vi "USG_Query HW.vi"(0 "System no.":i32=1 min=1 max=4 step=1, 5 "error in":errorcluster) -> (14 "List of Hardware Overview":string, 19 "error out":errorcluster)   [LabVIEW 2020]
doc: "USG? HW (Hardware Overview)\n\nDescription\nOutputs the \"HW\" section of the user guide. The \"HW\" section contains information on the \ncurrent hardware configuration and the associated firmware.\n\nFormat\nUSG? HW\n\nArguments\nnone\n\nResponse\nUSG? HW outputs a list of information on the hardware and firmware of the controller. The \nresponse consists of a block:\nThe HW block consists of at least the following fields:\n- Matchcode Match code of the hardware\n- Version Version of the hardware\n- Serial Number Serial number of the hardware\n- Date Production date of the hardware\nIn addition, the HW block contains at least the subblocks Dynamic HW and FW: \nThe Dynamic HW block consists of at least the following fields:\n- Property A property of the hardware, e.g. MAC address or vendor ID \n- Type Data type of the property value\n- Value Property value\nThe FW block consists of at least the following fields:\n- Container Unit Alias for the container unit to which the firmware belongs\n- Function Unit Alias for the function unit to which the firmware belongs\n- ID Index of the firmware in the controller\n- Matchcode Match code of the firmware\n- Version Version of the firmware\n- Date Date of the firmware\n- Compatibility Compatibility index\n- Description Short description of the firmware\n\nNotes\nUSG? HW is comparable to VER? (p. 81) and *IDN? (p. 7) from GCS 2.0, but not identical to \nthese commands.\n\nUser command level\nUSR"
panel:
  # "USG? HW (Hardware Overview)\n\nOutputs the \"HW\" section of the user guide. The \"HW\" section contains information on the \ncurrent hardware configuration and the associated firmware."
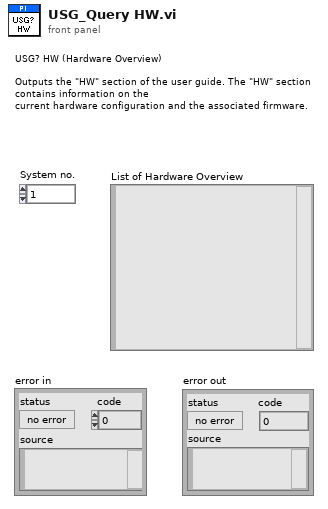
[diagram p1: front panel]
types:
  T1 = typedef "Syntax.ctl" = enum16{"GCS 1.0", "GCS 2.0", "GCS 3.0"}
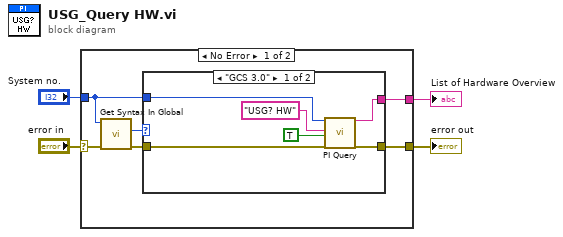
[diagram p0: block diagram]
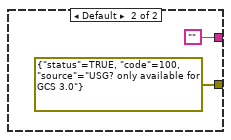
[diagram p2: hidden frame]
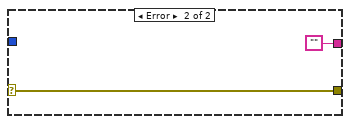
[diagram p3: hidden frame]
diagram:
  n1 = case shown="No Error" "error in" {
    selector: "error in" -> [w9 w20]
    tunnel: [w10 w20] -> w2
    tunnel: "System no." -> [w6 _]
    tunnel: [w5 ""] -> w1
    frame No Error {
      n2 = call "Get Syntax In Global.vi"("error in"=w9, "System no."=w6) -> ("error out"=w8:errorcluster, "Syntax"=w7:T1)  [unwired: 8 in]
      n3 = case shown="\"GCS 3.0\"" w7 {
        tunnel: [w11 errorcluster {"status"=TRUE, "code"=100, "source"="USG? only available for GCS 3.0"} ("error out")] -> w10
        tunnel: w6 -> [w16 _]
        tunnel: w8 -> [w15 _]
        tunnel: [w12 ""] -> w5
        frame "GCS 3.0" {
          n4 = call "PI Query.vi"("System no."=w16, "String to send"="USG? HW", "Attach termination char.?"=TRUE, "error in"=w15) -> ("String read"=w12:string, "error out"=w11:errorcluster)  [unwired: 12 in, 2 out]
        }
        frame Default {
        }
      }
    }
    frame Error {
    }
  }
  "error out" <- w2
  "List of Hardware Overview" <- w1
